vi "Read Icon.vi"(8 "error in (no error)":errorcluster, 11 "Icon in":refnum<class "Icon.lvclass">) -> (0 "error out":errorcluster, 2 "Icon":refnum<k24>, 3 "Icon out":refnum<class "Icon.lvclass">)   [LabVIEW 2016, in "Icon.lvclass"]
uses:
  Icon.lvclass
  System.Drawing
  Icon.lvclass/Icon.ctl
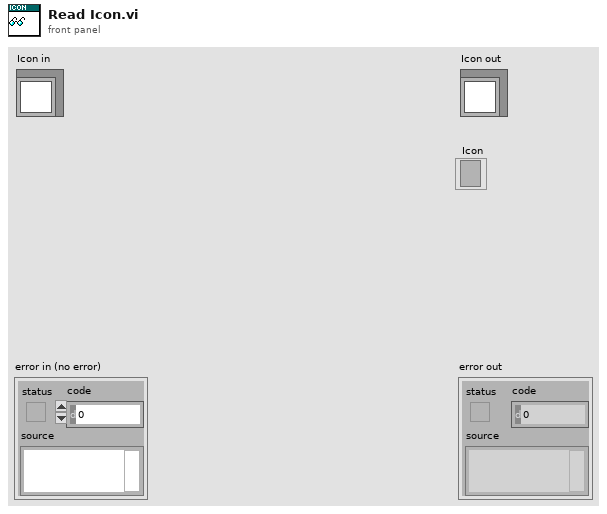
[diagram p1: front panel]
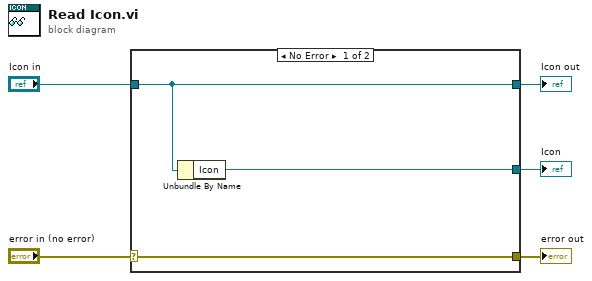
[diagram p0: block diagram]
diagram:
  n1 = case shown="No Error" "error in (no error)" {
    selector: "error in (no error)" -> [w8 w9]
    tunnel: [w8 w9] -> w4
    tunnel: [w7 w10] -> w2
    tunnel: "Icon in" -> [w7 w10]
    tunnel: [w6 _] -> w1
    frame No Error {
      n2 = Unbundle By Name(w7) -> ("Icon"=w6:refnum<k24>)
    }
    frame Error {
    }
  }
  "error out" <- w4
  "Icon out" <- w2
  "Icon" <- w1
